vi "modbus.vi"() -> ()   [LabVIEW 2019]
panel:
  in  "command":string="04"
  out "hex integer string":string
  in  "Set Points":dbl[](array[numeric])
  # ":010400000002F9"
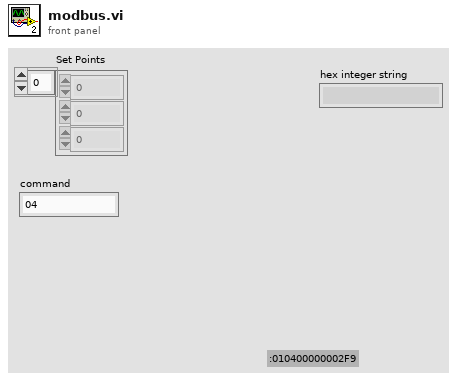
[diagram p1: front panel]
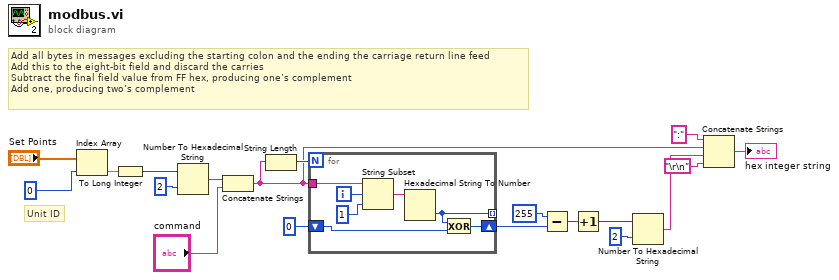
[diagram p0: block diagram]
diagram:
  # "Add all bytes in messages excluding the starting colon and the ending the carriage return line feed\nAdd this to the eight-bit field and discard the carries\nSubtract the final field value from FF hex, producing one’s complement\nAdd one, producing two’s complement"
  # "Unit ID"
  n1 = Index Array(array="Set Points", index=0) -> (element=w17:dbl)
  n2 = To Long Integer(number=w17) -> (32bit integer=w16:i32)
  n3 = Number To Hexadecimal String(1:i16 2 ("width (-)"), 2:w16) -> (0:w13:string)
  n4 = Concatenate Strings(w13, "command") -> (w2:string)
  n5 = String Length(string=w2) -> (length=w8:i32)
  n6 = for {
    N: w8 -> [_]
    tunnel: w2 -> [w23]
    shift-right: [w25] -> w1
    shift-left: u8 0 -> [w26]
    tunnel: [w24] -> _ mode=indexing
    i -> [w22]
    n7 = String Subset(string=w23, offset (0)=w22, length (rest)=1 ("length (rest)")) -> (substring=w20:string)
    n8 = Hexadecimal String To Number(string=w20) -> (number=w24:u32)  [unwired: 2 in, 1 out]
    n9 = Exclusive Or(1:w26, 2:w24) -> (0:w25:u32)
  }
  n10 = Subtract(x=255, y=w1) -> (x-y=w6:u32)
  n11 = Increment(x=w6) -> (x+1=w5:u32)
  n12 = Number To Hexadecimal String(1:i16 2 ("width (-)"), 2:w5) -> (0:w3:string)
  n13 = Concatenate Strings(":" ("string"), w2, w3, "\r\n") -> (→"hex integer string":string)
